vi "ListAutoPath.vi"() -> (2 "AutoRoutinesNames":string[](array[string]))   [LabVIEW 2023]
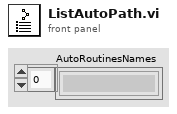
[diagram p1: front panel]
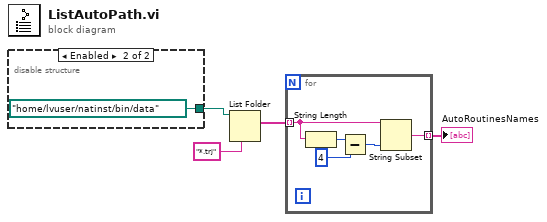
[diagram p0: block diagram]
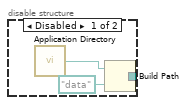
[diagram p2: hidden frame]
diagram:
  n1 = disable-structure shown="Enabled" {
    disable-tunnel: [w5 path "/home/lvuser/natinst/bin/data" ("appended path")] -> w4
    frame Disabled {
      n2 = call <vilib>:"Application Directory.vi"() -> ("Application Directory"=w7:path)
      n3 = Build Path(base path=w7, name or relative path=path "data") -> (appended path=w5:path)
    }
    frame Enabled {
    }
  }
  n4 = List Folder(path=w4, pattern="*.trj") -> (filenames=w2:string[])  [unwired: 2 in, 3 out]
  n5 = for {
    tunnel: w2 -> [w13] mode=indexing
    tunnel: [w9] -> w1 mode=indexing
    n6 = String Length(string=w13) -> (length=w12:i32)
    n7 = Subtract(x=w12, y=4) -> (x-y=w11:i32)
    n8 = String Subset(string=w13, length (rest)=w11) -> (substring=w9:string)  [unwired: 1 in]
  }
  "AutoRoutinesNames" <- w1
